vi "vTestStudioCfgEditor.vi"() -> ()   [LabVIEW 2010]
panel:
  out "Execution:State":T1(ring)=enum."Run top level"
  out "error out":errorcluster
  in  "error in":errorcluster
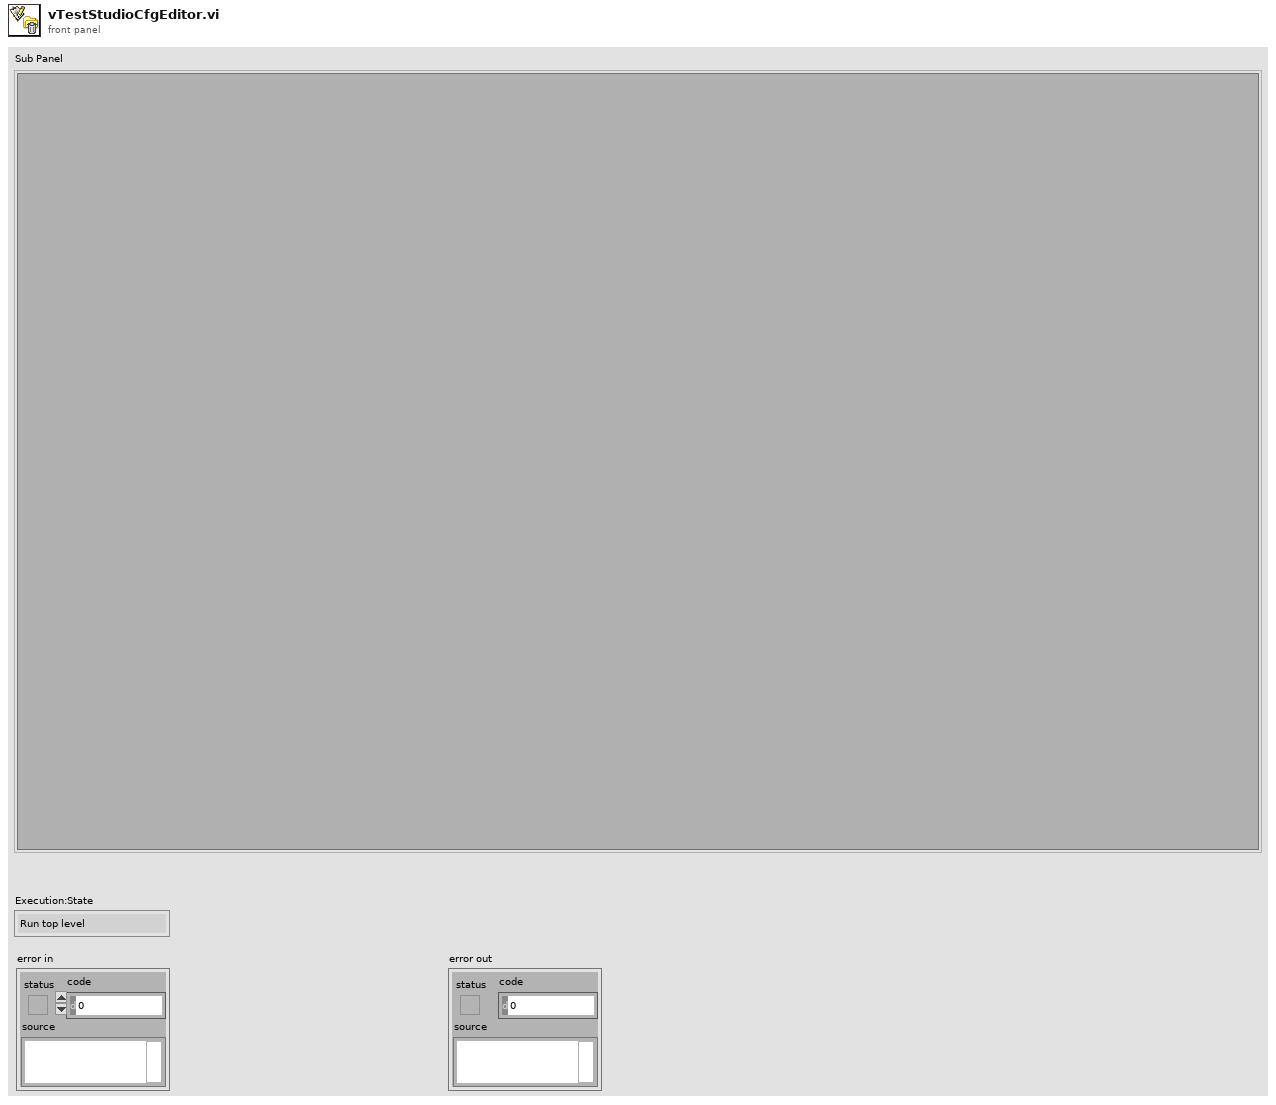
[diagram p1: front panel]
types:
  T1 = enum32{"Bad", "Idle", "Run top level", "Running"}
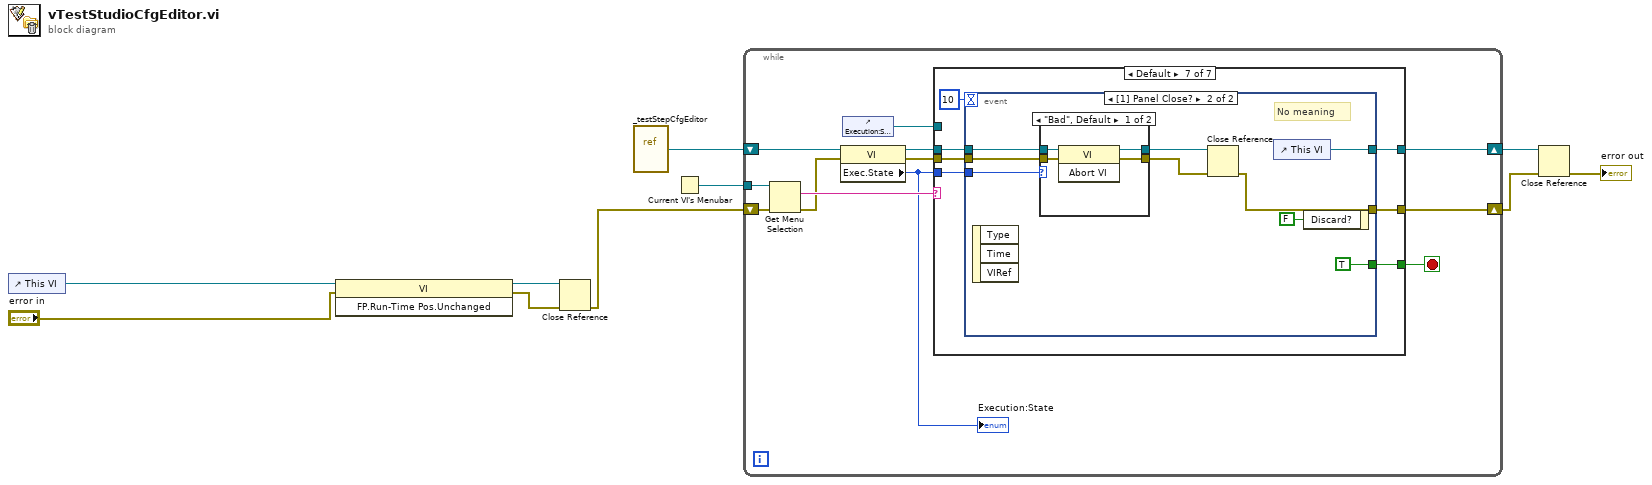
[diagram p0: block diagram]
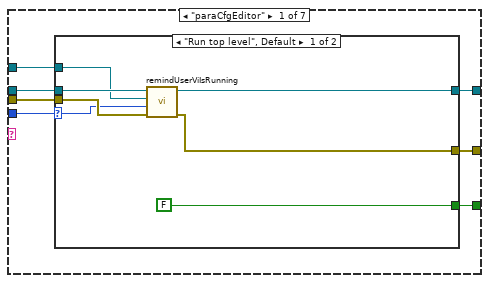
[diagram p2: hidden frame]
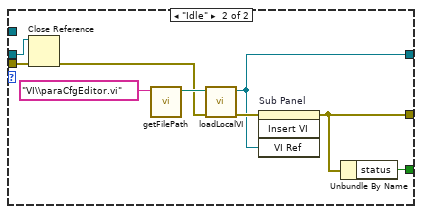
[diagram p3: hidden frame]
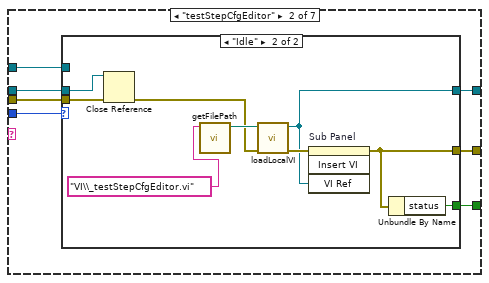
[diagram p4: hidden frame]
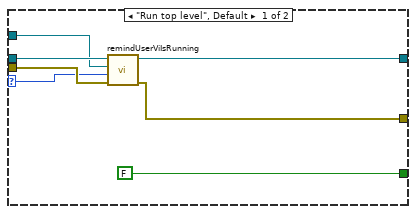
[diagram p5: hidden frame]
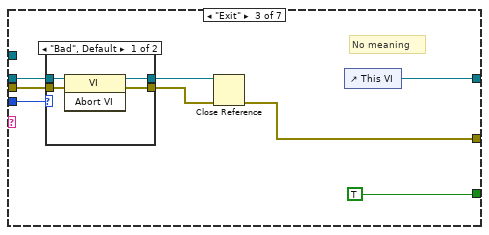
[diagram p6: hidden frame]
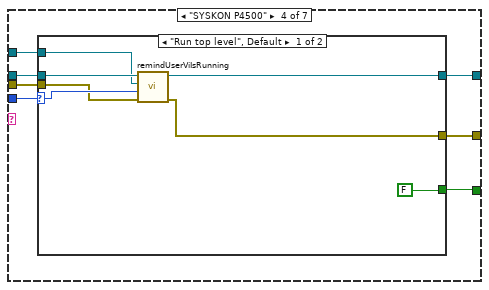
[diagram p8: hidden frame]
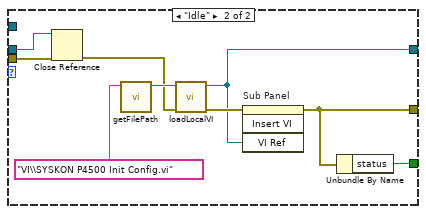
[diagram p9: hidden frame]
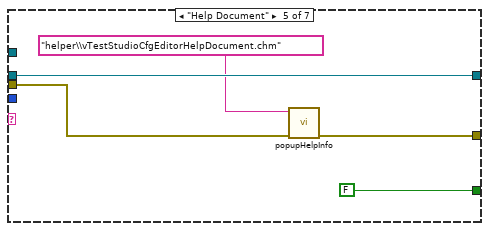
[diagram p10: hidden frame]
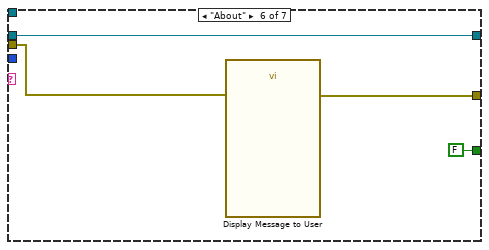
[diagram p11: hidden frame]
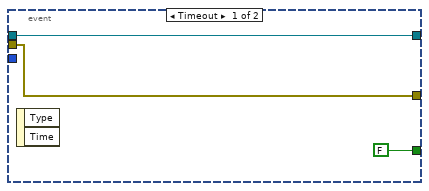
[diagram p12: hidden frame]
diagram:
  n1 = control-ref of="This VI"() -> (w5:refnum<vi>)
  n2 = invoke class="VI" method="FP.Run-Time Pos.Unchanged"(reference=w5, error in="error in") -> (reference out=w8:refnum<vi>, error out=w7:errorcluster)  [unwired: 1 in, 1 out]
  n3 = Close Reference(reference=w8, error in (no error)=w7) -> (error out=w6:errorcluster)
  n4 = vi-ref "_testStepCfgEditor.vi"() -> (w9:refnum<vi>)
  n5 = Current VI's Menubar() -> (w10:refnum<k9>)
  n6 = while {
    tunnel: w10 -> [w22]
    shift-right: [w20] -> w2
    shift-left: w6 -> [w19]
    shift-right: [w17] -> w3
    shift-left: w9 -> [w16]
    stop <- w18 stop-if-true
    n7 = Get Menu Selection(0:w22, 3:w19) -> (6:w21:string, 8:w12:errorcluster)  [unwired: 2 in, 3 out]
    n8 = property class="VI"(reference=w16, error in=w12) -> (reference out=w15:refnum<vi>, error out=w14:errorcluster, "Exec.State"=w11:T1)
    "Execution:State" <- w11
    n9 = control-ref of="Execution:State"() -> (w13:refnum<vi>)
    n10 = case shown="Default" w21 {
      tunnel: [w28 w47 w75 w87 w107 w111 w119] -> w20
      tunnel: [w29 w46 TRUE w86 FALSE FALSE ("status") w117] -> w18
      tunnel: [w27 w48 w74 w85 w109 w114 w118] -> w17
      tunnel: w15 -> [w26 w52 w73 w89 w109 w114 w121]
      tunnel: w14 -> [w25 w51 w72 w88 w108 w112 w120]
      tunnel: w11 -> [w24 w50 w69 w84 _ _ w116]
      tunnel: w13 -> [w23 w49 _ w83 _ _ _]
      frame "paraCfgEditor" {
        n11 = case shown="\"Run top level\", Default" w24 {
          selector: w24 -> [w30 _]
          tunnel: [FALSE ("status") w45] -> w29
          tunnel: [w32 w44] -> w28
          tunnel: [w33 w40] -> w27
          tunnel: w25 -> [w34 w42]
          tunnel: w26 -> [w35 w41]
          tunnel: w23 -> [w31 _]
          frame "Run top level", Default {
            n12 = call "remindUserViIsRunning.vi"("error in"=w34, "enumIndex"=w30, "Enum Refnum"=w31, "VI reference in"=w35) -> ("error out"=w32:errorcluster, "VI reference out"=w33:refnum<vi>)  [unwired: 6 in]
          }
          frame "Idle" {
            n13 = Close Reference(reference=w41, error in (no error)=w42) -> (error out=w37:errorcluster)
            n14 = call "getFilePath.vi"("fileName"="VI\\paraCfgEditor.vi") -> ("path"=w39:path)  [unwired: 10 in]
            n15 = call "loadLocalVI.vi"("error in"=w37, "vi path"=w39) -> ("error out"=w43:errorcluster, "vi reference"=w40:refnum<vi>)  [unwired: 8 in]
            n16 = invoke on="Sub Panel" class="SubPanel" method="Insert VI"(error in=w43, "VI Ref"=w40) -> (error out=w44:errorcluster)  [unwired: 2 in, 3 out]
            n17 = Unbundle By Name(w44) -> ("status"=w45:bool)
          }
        }
      }
      frame "testStepCfgEditor" {
        n18 = case shown="\"Idle\"" w50 {
          selector: w50 -> [w53 _]
          tunnel: [FALSE ("status") w68] -> w46
          tunnel: [w55 w67] -> w47
          tunnel: [w56 w63] -> w48
          tunnel: w51 -> [w57 w65]
          tunnel: w52 -> [w58 w64]
          tunnel: w49 -> [w54 _]
          frame "Run top level", Default {
            n19 = call "remindUserViIsRunning.vi"("error in"=w57, "enumIndex"=w53, "Enum Refnum"=w54, "VI reference in"=w58) -> ("error out"=w55:errorcluster, "VI reference out"=w56:refnum<vi>)  [unwired: 6 in]
          }
          frame "Idle" {
            n20 = Close Reference(reference=w64, error in (no error)=w65) -> (error out=w60:errorcluster)
            n21 = call "getFilePath.vi"("fileName"="VI\\_testStepCfgEditor.vi") -> ("path"=w62:path)  [unwired: 10 in]
            n22 = call "loadLocalVI.vi"("error in"=w60, "vi path"=w62) -> ("error out"=w66:errorcluster, "vi reference"=w63:refnum<vi>)  [unwired: 8 in]
            n23 = invoke on="Sub Panel" class="SubPanel" method="Insert VI"(error in=w66, "VI Ref"=w63) -> (error out=w67:errorcluster)  [unwired: 2 in, 3 out]
            n24 = Unbundle By Name(w67) -> ("status"=w68:bool)
          }
        }
      }
      frame "Exit" {
        # "No meaning"
        n25 = case shown="\"Bad\", Default" w69 {
          tunnel: w73 -> [w80 w82]
          tunnel: w72 -> [w79 w81]
          tunnel: [w78 w82] -> w71
          tunnel: [w77 w81] -> w70
          frame "Bad", Default {
            n26 = invoke class="VI" method="Abort VI"(reference=w80, error in=w79) -> (reference out=w78:refnum<vi>, error out=w77:errorcluster)  [unwired: 1 in, 1 out]
          }
          frame "Idle" {
          }
        }
        n27 = Close Reference(reference=w71, error in (no error)=w70) -> (error out=w75:errorcluster)
        n28 = control-ref of="This VI"() -> (w74:refnum<vi>)
      }
      frame "SYSKON P4500" {
        n29 = case shown="\"Run top level\", Default" w84 {
          selector: w84 -> [w94 _]
          tunnel: w89 -> [w96 w105]
          tunnel: w88 -> [w93 w104]
          tunnel: [w92 w103] -> w87
          tunnel: [FALSE ("status") w102] -> w86
          tunnel: [w91 w97] -> w85
          tunnel: w83 -> [w95 _]
          frame "Run top level", Default {
            n30 = call "remindUserViIsRunning.vi"("error in"=w93, "enumIndex"=w94, "Enum Refnum"=w95, "VI reference in"=w96) -> ("error out"=w92:errorcluster, "VI reference out"=w91:refnum<vi>)  [unwired: 6 in]
          }
          frame "Idle" {
            n31 = Close Reference(reference=w105, error in (no error)=w104) -> (error out=w98:errorcluster)
            n32 = call "getFilePath.vi"("fileName"="VI\\SYSKON P4500 Init Config.vi") -> ("path"=w100:path)  [unwired: 10 in]
            n33 = call "loadLocalVI.vi"("error in"=w98, "vi path"=w100) -> ("error out"=w101:errorcluster, "vi reference"=w97:refnum<vi>)  [unwired: 8 in]
            n34 = invoke on="Sub Panel" class="SubPanel" method="Insert VI"(error in=w101, "VI Ref"=w97) -> (error out=w103:errorcluster)  [unwired: 2 in, 3 out]
            n35 = Unbundle By Name(w103) -> ("status"=w102:bool)
          }
        }
      }
      frame "Help Document" {
        n36 = call "popupHelpInfo.vi"("error in"=w108, "fileName"="helper\\vTestStudioCfgEditorHelpDocument.chm") -> ("error out"=w107:errorcluster)  [unwired: 9 in]
      }
      frame "About" {
        n37 = call "Display Message to User"("error in (no error)"=w112) -> ("error out"=w111:errorcluster)  [unwired: 9 in, 1 out]
      }
      frame Default {
        n38 = event shown="[1] Panel Close?" {
          selector: _ -> [_ _]
          dyn-events: _ -> [_ _]
          timeout: 10 -> [_ _]
          tunnel: w121 -> [w123 w131]
          tunnel: w120 -> [w124 w130]
          tunnel: [w124 w129] -> w119
          tunnel: [w123 w128] -> w118
          tunnel: [FALSE TRUE] -> w117
          tunnel: w116 -> [_ w126]
          event Timeout {
            n39 = event-data() -> ()  [unwired: 1 in, 2 out]
          }
          event Panel Close? {
            # "No meaning"
            n40 = event-data() -> ()  [unwired: 1 in, 3 out]
            n41 = case shown="\"Bad\", Default" w126 {
              tunnel: w131 -> [w137 w139]
              tunnel: w130 -> [w136 w138]
              tunnel: [w135 w139] -> w133
              tunnel: [w134 w138] -> w132
              frame "Bad", Default {
                n42 = invoke class="VI" method="Abort VI"(reference=w137, error in=w136) -> (reference out=w135:refnum<vi>, error out=w134:errorcluster)  [unwired: 1 in, 1 out]
              }
              frame "Idle" {
              }
            }
            n43 = Close Reference(reference=w133, error in (no error)=w132) -> (error out=w129:errorcluster)
            n44 = control-ref of="This VI"() -> (w128:refnum<vi>)
            n45 = event-data("Discard?"=FALSE) -> ()  [unwired: 1 in, 1 out]
          }
        }
      }
    }
  }
  n46 = Close Reference(reference=w3, error in (no error)=w2) -> (error out=→"error out":errorcluster)
